vi "Get Initial FP Control Positions.vi"(8 "error in (no error)":errorcluster, 10 "Pane":refnum<vi>, 11 "AppMgr in":refnum<class "Application Manager.lvclass">) -> (0 "error out":errorcluster, 3 "AppMgr out":refnum<class "Application Manager.lvclass">)   [LabVIEW 2017, in "Application Manager.lvclass"]
doc: "Get the initial positons of resizable front panel elements"
uses:
  Application Manager.lvclass
  Application Manager.lvclass/Application Manager.ctl
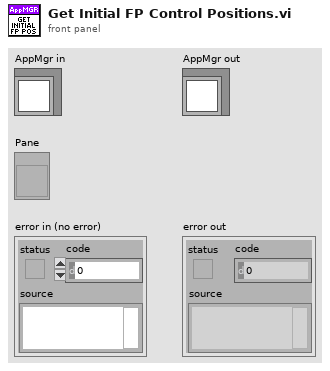
[diagram p1: front panel]
types:
  T1 = typedef "LVBoundsTypeDef.ctl" = cluster{"Width":u32, "Height":u32}
  T2 = typedef "LVPositionTypeDef.ctl" = cluster{"Left":i32, "Top":i32}
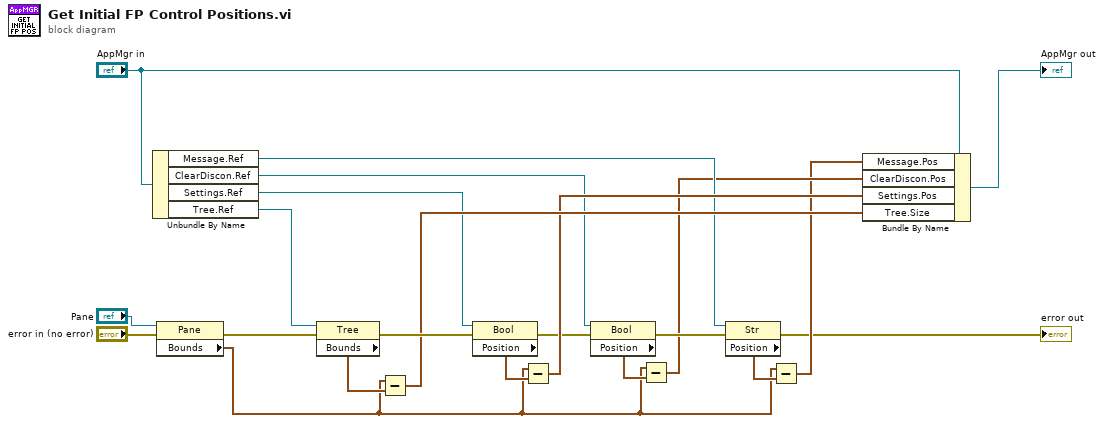
[diagram p0: block diagram]
diagram:
  n1 = Unbundle By Name("AppMgr in") -> ("Message.Ref"=w5:refnum<vi>, "ClearDiscon.Ref"=w6:refnum<vi>, "Settings.Ref"=w12:refnum<vi>, "Tree.Ref"=w16:refnum<vi>)
  n2 = property class="Pane"(reference="Pane", error in="error in (no error)") -> (error out=w15:errorcluster, "Bounds"=w4:T1)  [unwired: 1 out]
  n3 = property class="Tree"(reference=w16, error in=w15) -> (error out=w14:errorcluster, "Bounds"=w17:T1)  [unwired: 1 out]
  n4 = Subtract(x=w4, y=w17) -> (x-y=w13:T1)
  n5 = property class="Bool"(reference=w12, error in=w14) -> (error out=w7:errorcluster, "Position"=w22:T2)  [unwired: 1 out]
  n6 = Subtract(x=w4, y=w22) -> (x-y=w11:T1)
  n7 = property class="Bool"(reference=w6, error in=w7) -> (error out=w8:errorcluster, "Position"=w10:T2)  [unwired: 1 out]
  n8 = Subtract(x=w4, y=w10) -> (x-y=w3:T1)
  n9 = property class="Str"(reference=w5, error in=w8) -> (error out=→"error out":errorcluster, "Position"=w9:T2)  [unwired: 1 out]
  n10 = Subtract(x=w4, y=w9) -> (x-y=w2:T1)
  n11 = Bundle By Name(cluster="AppMgr in", "Message.Pos"=w2, "ClearDiscon.Pos"=w3, "Settings.Pos"=w11, "Tree.Size"=w13) -> (→"AppMgr out":refnum<class "Application Manager.lvclass">)
